vi "Create Message Queue.vi"(8 "error in (no error)":errorcluster, 10 "Max Size (1000)":i32=1000, 11 "Queue Name":string) -> (0 "error out":errorcluster, 3 "queue out":refnum<queue>)   [LabVIEW 2019, in "Messaging.lvlib"]
doc: "Create and preallocate memory for queue elements.\n\nInfinite sized queues (-1) do not have memory preallocated."
uses:
  Messaging.lvlib
  Message Cluster.ctl
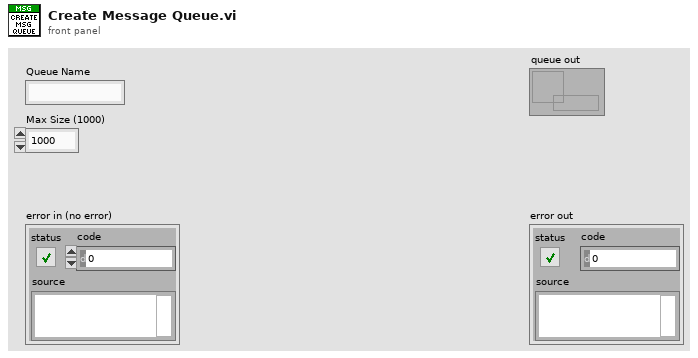
[diagram p1: front panel]
types:
  T1 = typedef "Messaging.lvlib/Message Cluster.ctl" = cluster{"Event":string, "Source":string, "Target":string, "Data":variant}
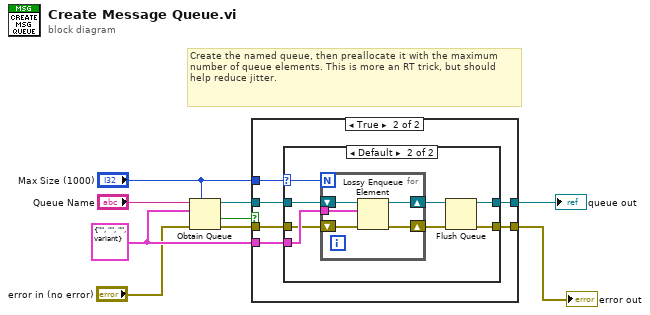
[diagram p0: block diagram]
diagram:
  w9 = T1 {"Event"="", "Source"="", "Target"="", "Data"=variant} ("Message")
  # "Create the named queue, then preallocate it with the maximum number of queue elements. This is more an RT trick, but should help reduce jitter."
  n1 = Obtain Queue(max queue size (-1, unlimited)="Max Size (1000)", name (unnamed)="Queue Name", element data type=w9, error in (no error)="error in (no error)") -> (queue out=w7:refnum<queue>, created new?=w1:bool, error out=w3:errorcluster)  [unwired: 1 in]
  n2 = case shown="True" w1 {
    tunnel: w9 -> [_ w17]
    tunnel: "Max Size (1000)" -> [_ w12]
    tunnel: w7 -> [w11 w16]
    tunnel: [w11 w15] -> w5
    tunnel: w3 -> [w10 w14]
    tunnel: [w10 w13] -> w2
    frame False {
    }
    frame True {
      n3 = case shown="Default" w12 {
        selector: w12 -> [_ w20]
        tunnel: w17 -> [_ w26]
        tunnel: w16 -> [w19 w25]
        tunnel: [w19 w24] -> w15
        tunnel: w14 -> [w18 w23]
        tunnel: [w18 w21] -> w13
        frame ..-1 {
          # "Don't try fill an infinite queue"
        }
        frame Default {
          n4 = for {
            N: w20 -> [_]
            shift-right: [w31] -> w27
            shift-left: w25 -> [w32]
            tunnel: w26 -> [w30]
            shift-right: [w28] -> w22
            shift-left: w23 -> [w29]
            n5 = Lossy Enqueue Element(queue=w32, element=w30, error in (no error)=w29) -> (queue out=w31:refnum<queue>, error out=w28:errorcluster)  [unwired: 2 out]
          }
          n6 = Flush Queue(queue=w27, error in (no error)=w22) -> (queue out=w24:refnum<queue>, error out=w21:errorcluster)  [unwired: 1 out]
        }
      }
    }
  }
  "queue out" <- w5
  "error out" <- w2
